vi "Ophir InitCom-AutoFind.vi"(4 "Baud Rate (3:9600)":i16(ring)=4 items=["300", "1200", "4800", "9600", "19200", "38400"], 5 "communication":i16(ring) items=["USB - Nova2", "USB - Vega", "USB - USBI", "RS232", "GPIB"], 6 "Port Number (default 2)":i16=1 min=0 max=20, 7 "error in (no error)":errorcluster) -> (0 "Dup Visa Session":refnum<visa-resource-name>, 1 "Ophir Board":string, 2 "Debug Index":i32, 3 "error out":errorcluster)   [LabVIEW 2012]
doc: "InitCom.vi initializes the communication with Nova2 and\nreturns the VISA Session. \nVersion 1.00 \nLast Updated 16 Mars 2005\n\nYou must run this VI before using any of the instrument driver VIs for this instrument.\n\nYou must choose Communication Protocol : USB or RS232\nwhen USB is default.\n\nFor RS232 Protocol you must fill the Port Number and the Baud Rate.\n\nInputs:\nUSB/RS232:Boolean\nSelect Protocol USB(True) or RS232(False)\nDefault True:USB\n\nDevice Address:\nString defaut:10 for Nova2 Device\nPort Number\nThe Port Number control specifies the serial port .\nPort Number 1 corresponds to serial port 1, Port Number 2 = serial port 2, etc.\ndefault: 2\n\nBaud Rate :\n0:300 bps\n1:1200 bps\n2:4800 bps\n3:9600 bps\n4:19200 bps\n5:38400 bps\ndefault: 3:9600 bps\n\nOutputs:\ndup Visa Session\nErrorOut\n\nNote:\nThe Device fixed communication parameters are:\nData bits:8\nStop bits:1\nParity:None"
panel:
  out "Visa Session":refnum<visa-resource-name>
  # "PC:  1 = COM1, 2= COM2,.."
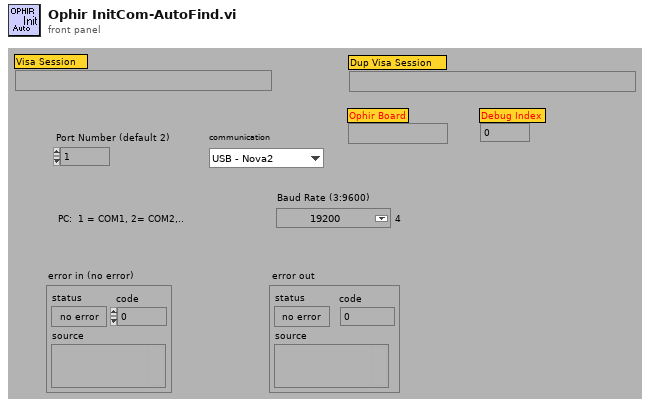
[diagram p1: front panel]
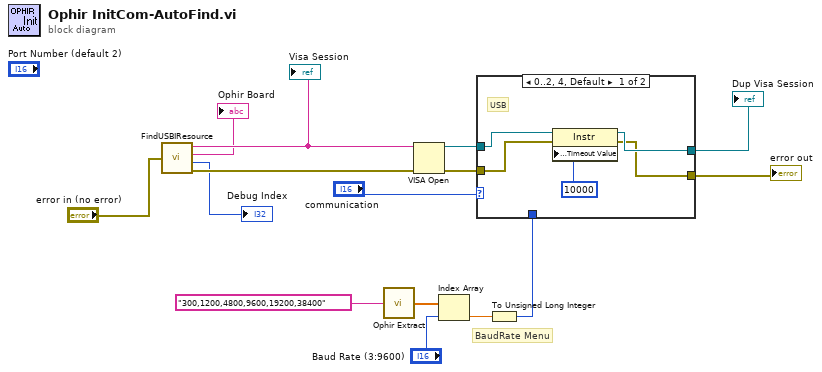
[diagram p0: block diagram]
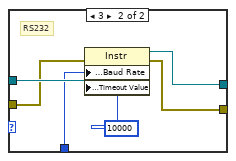
[diagram p2: hidden frame]
diagram:
  # "BaudRate Menu"
  n1 = call "FindUSBIResource.vi"("error in (no error)"="error in (no error)") -> ("Ophir Resource"=w3:string, "Ophir Board"=→"Ophir Board":string, "Debug Index"=→"Debug Index":i32, "error out"=w4:errorcluster)
  "Visa Session" <- w3
  n2 = call "Ophir Extract.vi"("String"="300,1200,4800,9600,19200,38400") -> ("Single Precision Array"=w10:sgl[])
  n3 = VISA Open(error in (no error)=w4, VISA resource name=w3) -> (VISA resource name=w15:refnum<visa-resource-name>, error out=w12:errorcluster)  [unwired: 3 in]
  n4 = Index Array "Index Array"(array=w10, index="Baud Rate (3:9600)") -> (element=w8:sgl)
  n5 = To Unsigned Long Integer(number=w8) -> (unsigned 32bit integer=w7:u32)
  n6 = case shown="0..2, 4, Default" "communication" {
    tunnel: w15 -> [w20 w26]
    tunnel: [w19 w25] -> w14
    tunnel: [w17 w23] -> w13
    tunnel: w12 -> [w18 w24]
    tunnel: w7 -> [_ w22]
    frame 0..2, 4, Default {
      # "USB"
      n7 = property class="Instr"(reference=w20, error in=w18, "General Settings:Timeout Value"=u32 10000) -> (reference out=w19:refnum<visa-resource-name>, error out=w17:errorcluster)
    }
    frame 3 {
      # "RS232"
      n8 = property class="Instr"(reference=w26, error in=w24, "Serial Settings:Baud Rate"=w22, "General Settings:Timeout Value"=u32 10000) -> (reference out=w25:refnum<visa-resource-name>, error out=w23:errorcluster)
    }
  }
  "error out" <- w13
  "Dup Visa Session" <- w14
